vi "LowLvGV.vi"() -> ()   [LabVIEW 2015]
panel:
  in  "MTP Folder":path=path "c:/AKM43L_Param"
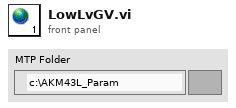
[diagram p1: front panel]
diagram:
